vi "PipBoy_RemoveFromQIfExist.vi"(8 "error in (no error)":errorcluster, 10 "Message":string="AcquirePipBoy", 11 "Message Queue":refnum<queue>) -> (0 "error out":errorcluster)   [LabVIEW 2014]
uses:
  modules/support/Message Queue/Message Cluster.ctl
  modules/support/Message Queue/Message Queue.lvlib
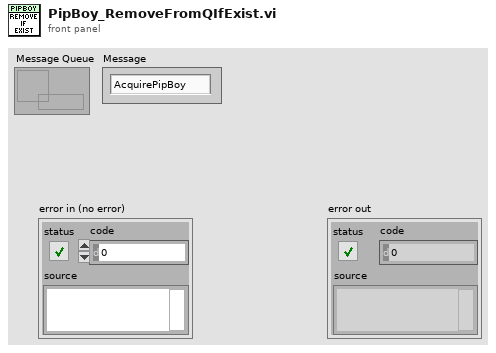
[diagram p1: front panel]
types:
  T1 = typedef "Message Queue.lvlib/Message Cluster.ctl" = cluster{"Message":string, "Message Data":variant}
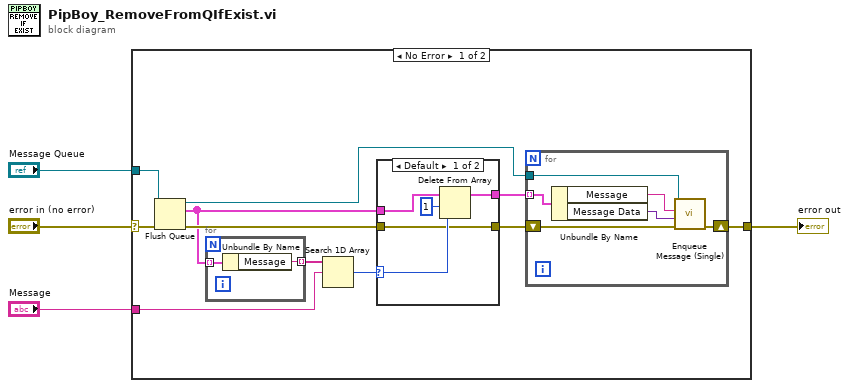
[diagram p0: block diagram]
diagram:
  n1 = case shown="No Error" "error in (no error)" {
    selector: "error in (no error)" -> [w10 w31]
    tunnel: "Message Queue" -> [w15 _]
    tunnel: [w7 w31] -> w3
    tunnel: "Message" -> [w13 _]
    frame No Error {
      n2 = Flush Queue(queue=w15, error in (no error)=w10) -> (queue out=w5:refnum<queue>, remaining elements=w9:T1[], error out=w11:errorcluster)
      n3 = for {
        tunnel: w9 -> [w23] mode=indexing
        tunnel: [w22] -> w14 mode=indexing
        n4 = Unbundle By Name(w23) -> ("Message"=w22:string)
      }
      n5 = Search 1D Array(1D array=w14, element=w13) -> (index of element=w12:i32)  [unwired: 1 in]
      n6 = case shown="Default" w12 {
        selector: w12 -> [w26 _]
        tunnel: w11 -> [w25 w30]
        tunnel: [w25 w30] -> w8
        tunnel: w9 -> [w28 w29]
        tunnel: [w24 w29] -> w6
        frame Default {
          n7 = Delete From Array(array=w28, length=1, index=w26) -> (array with subset deleted=w24:T1[])  [unwired: 1 out]
        }
        frame -1 {
        }
      }
      n8 = for {
        tunnel: w6 -> [w18] mode=indexing
        shift-right: [w20] -> w7
        shift-left: w8 -> [w21]
        tunnel: w5 -> [w19]
        n9 = Unbundle By Name(w18) -> ("Message"=w17:string, "Message Data"=w16:variant)
        n10 = call "Enqueue Message (Single).vi"("error in (no error)"=w21, "Message Data"=w16, "Message"=w17, "Message Queue"=w19) -> ("error out"=w20:errorcluster)  [unwired: 6 in, 1 out]
      }
    }
    frame Error {
    }
  }
  "error out" <- w3
